vi "CFD_scan.vi"(9 "Delay":dbl, 10 "Attenuation":dbl, 11 "Wvfm":waveform(dbl)[](array[waveform])) -> (0 "spectrum":i32[][](array[numeric]), 2 "min index(es)":i32[](array[numeric]), 3 "min value":dbl, 4 "Variables":cluster{"Attenuation":dbl, "Delay":dbl}[](array[cluster]))   [LabVIEW 2019]
uses:
  SiPM_Tests_Global_Var.vi
panel:
  out "Std_dev":dbl[][](array[numeric])
  out "Center":dbl[][](array[numeric])
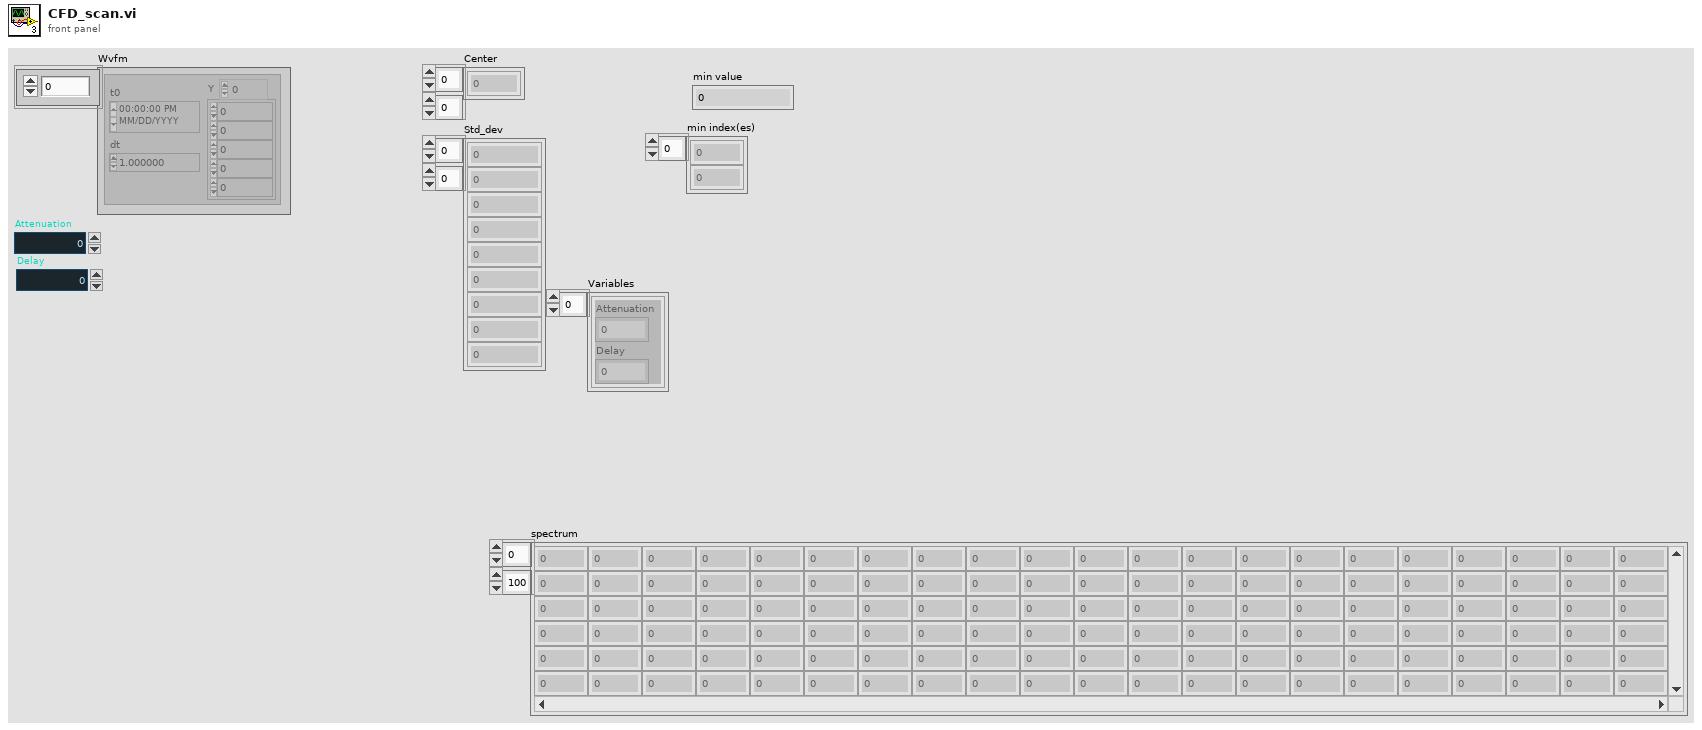
[diagram p1: front panel]
types:
  T1 = cluster{"Numeric Control":dbl, "center":dbl, "standard deviation":dbl, "amplitude":dbl}
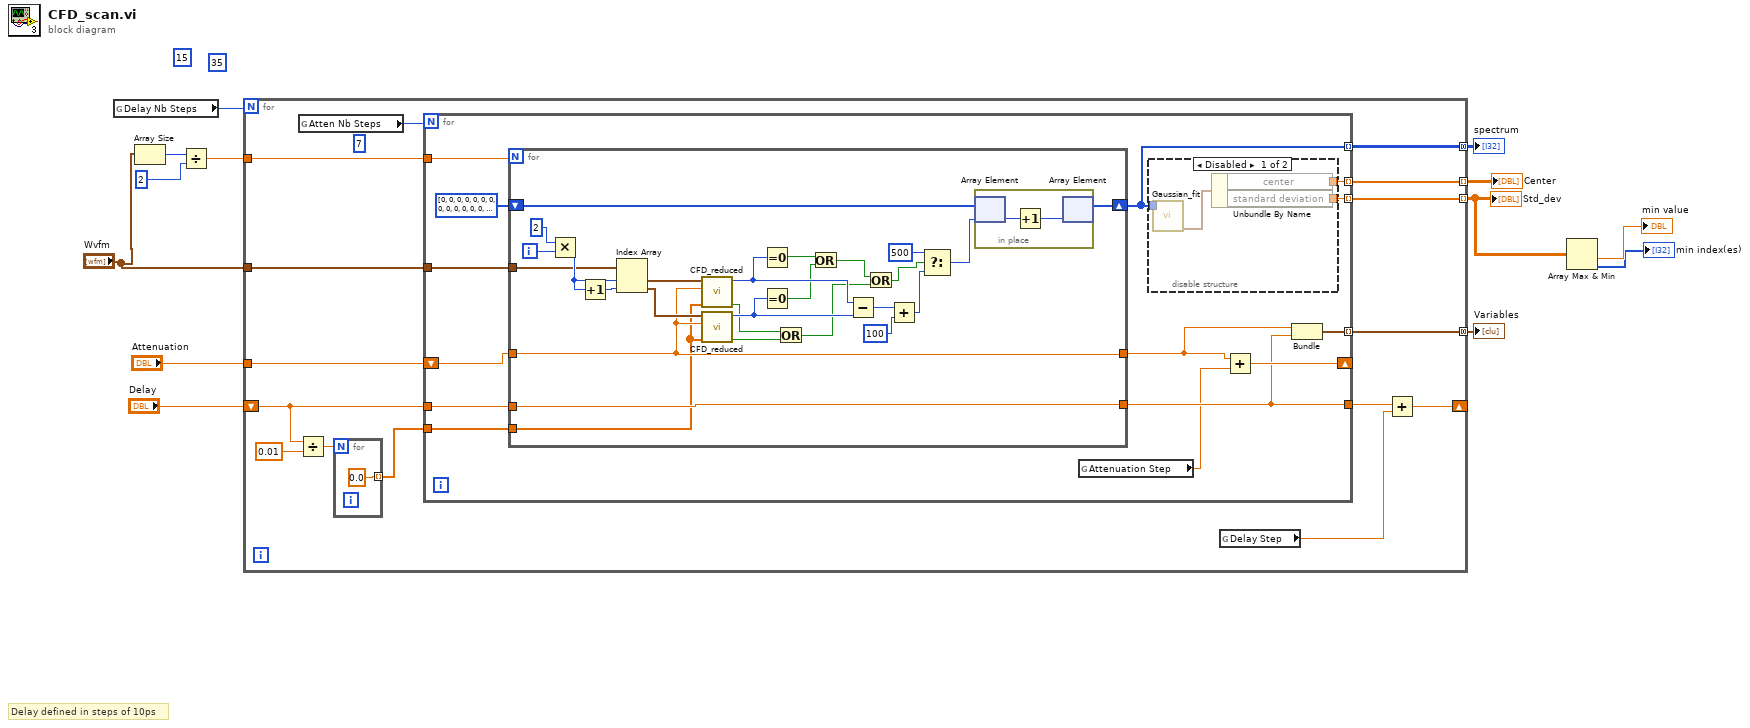
[diagram p0: block diagram]
diagram:
  (unwired) 15
  (unwired) 35
  # "Delay defined in steps of 10ps"
  n1 = global read "SiPM_Tests_Global_Var.vi" "Delay Nb Steps"() -> (w1:u8)
  n2 = Array Size(array="Wvfm") -> (size(s)=w12:i32)
  n3 = Divide(x=w12, y=2) -> (x/y=w9:dbl)
  n4 = for {
    N: w1 -> [_]
    tunnel: "Attenuation" -> [w28]
    tunnel: "Wvfm" -> [w27]
    tunnel: w9 -> [w26]
    shift-right: [w25] -> _
    shift-left: "Delay" -> [w18]
    tunnel: [w23] -> w7 mode=indexing
    tunnel: [w22] -> w6 mode=indexing
    tunnel: [w21] -> w3 mode=concatenating
    tunnel: [w16] -> w2 mode=concatenating
    (unwired) 7
    n5 = Divide(x=w18, y=0.01) -> (x/y=w20:dbl)
    n6 = global read "SiPM_Tests_Global_Var.vi" "Atten Nb Steps"() -> (w15:u8)
    n7 = for {
      N: w20 -> [_]
      tunnel: [0.0 ("new element/subarray")] -> w17 mode=indexing
    }
    n8 = for {
      N: w15 -> [_]
      tunnel: w27 -> [w42]
      tunnel: w26 -> [w41]
      shift-right: [w40] -> _
      shift-left: w28 -> [w43]
      tunnel: w18 -> [w39]
      tunnel: [w33] -> w24
      tunnel: [w37] -> w23 mode=indexing
      tunnel: [w36] -> w22 mode=indexing
      tunnel: [w35] -> w21 mode=indexing
      tunnel: w17 -> [w34]
      tunnel: [w31] -> w16 mode=indexing
      n9 = for {
        N: w41 -> [_]
        tunnel: w42 -> [w69]
        tunnel: w43 -> [w66]
        tunnel: [w66] -> w32
        tunnel: w39 -> [w61]
        tunnel: [w61] -> w33
        shift-right: [w62] -> w35
        shift-left: i32[] [0, 0, 0, 0, 0, 0, 0, 0, 0, 0, 0, 0, 0, 0, 0, 0, 0, 0, 0, 0, 0, 0, 0, 0, 0, 0, 0, 0, 0, 0, 0, 0, 0, 0, 0, 0, 0, 0, 0, 0, 0, 0, 0, 0, 0, 0, 0, 0, 0, 0, 0, 0, 0, 0, 0, 0, 0, 0, 0, 0, 0, 0, 0, 0, 0, 0, 0, 0, 0, 0, 0, 0, 0, 0, 0, 0, 0, 0, 0, 0, 0, 0, 0, 0, 0, 0, 0, 0, 0, 0, 0, 0, 0, 0, 0, 0, 0, 0, 0, 0, 0, 0, 0, 0, 0, 0, 0, 0, 0, 0, 0, 0, 0, 0, 0, 0, 0, 0, 0, 0, 0, 0, 0, 0, 0, 0, 0, 0, 0, 0, 0, 0, 0, 0, 0, 0, 0, 0, 0, 0, 0, 0, 0, 0, 0, 0, 0, 0, 0, 0, 0, 0, 0, 0, 0, 0, 0, 0, 0, 0, 0, 0, 0, 0, 0, 0, 0, 0, 0, 0, 0, 0, 0, 0, 0, 0, 0, 0, 0, 0, 0, 0, 0, 0, 0, 0, 0, 0, 0, 0, 0, 0, 0, 0, 0, 0, 0, 0, 0, 0, 0] ("Array") -> [w63]
        tunnel: w34 -> [w60]
        i -> [w68]
        n10 = Multiply(x=2, y=w68) -> (x*y=w71:i32)
        n11 = Increment(x=w71) -> (x+1=w73:i32)
        n12 = Index Array(array=w69, index #1=w71, index #2=w73) -> (element #1=w70:waveform(dbl), element #2=w67:waveform(dbl))
        n13 = call "CFD_reduced.vi"("Delay Array"=w60, "Attenuation"=w66, "Waveform_in"=w70) -> ("not_detected"=w51:bool, "CFD"=w59:i32)  [unwired: 7 in]
        n14 = call "CFD_reduced.vi"("Delay Array"=w60, "Attenuation"=w66, "Waveform_in"=w67) -> ("not_detected"=w52:bool, "CFD"=w58:i32)  [unwired: 7 in]
        n15 = Equal To 0?(x=w59) -> (x = 0?=w57:bool)
        n16 = Equal To 0?(x=w58) -> (x = 0?=w53:bool)
        n17 = Or(x=w51, y=w52) -> (x .or. y?=w49:bool)
        n18 = Or(x=w57, y=w53) -> (x .or. y?=w50:bool)
        n19 = Subtract(x=w59, y=w58) -> (x-y=w65:i32)
        n20 = Or(x=w50, y=w49) -> (x .or. y?=w48:bool)
        n21 = Add(x=w65, y=100) -> (x+y=w56:i32)
        n22 = Select(t=500, s=w48, f=w56) -> (s? t:f=w55:i32)
        n23 = in-place {
          n24 = in-place-array #1(w63, w55) -> (w75:i32)
          n25 = Increment(x=w75) -> (x+1=w74:i32)
          n26 = in-place-array #1(w74) -> (w62:i32[])  [unwired: 1 out]
        }
      }
      n27 = global read "SiPM_Tests_Global_Var.vi" "Attenuation Step"() -> (w30:dbl)
      n28 = disable-structure shown="Disabled" {
        disable-tunnel: [w46 _] -> w37
        disable-tunnel: [w45 _] -> w36
        disable-tunnel: w35 -> [w44 _]
        frame Disabled {
          n29 = call "Gaussian_fit.vi"("Input waveform"=w44) -> ("Fit cluster"=w47:T1)  [unwired: 5 in, 1 out]
          n30 = Unbundle By Name(w47) -> ("center"=w46:dbl, "standard deviation"=w45:dbl)
        }
        frame Enabled {
        }
      }
      n31 = Add(x=w32, y=w30) -> (x+y=w40:dbl)
      n32 = Bundle("Attenuation"=w32, "Delay"=w33) -> (w31:cluster{"Attenuation":dbl, "Delay":dbl})  [unwired: 1 in]
    }
    n33 = global read "SiPM_Tests_Global_Var.vi" "Delay Step"() -> (w14:dbl)
    n34 = Add(x=w24, y=w14) -> (x+y=w25:dbl)
  }
  "Center" <- w7
  "Std_dev" <- w6
  "spectrum" <- w3
  "Variables" <- w2
  n35 = Array Max & Min(array=w6) -> (min value=→"min value":dbl, min index (indices)=→"min index(es)":i32[])  [unwired: 2 out]
